vi "test bench_FXP_Linear_controller_observer.vi"() -> ()   [LabVIEW 2017]
uses:
  fixed-point/typeDefs/FXPControlParams_distEst.ctl
  fixed-point/typeDefs/x_vec_bram.ctl
  fixed-point/typeDefs/Kz_bram.ctl
  fixed-point/typeDefs/Nx_bram.ctl
  fixed-point/typeDefs/A_as_vec_bram.ctl
  fixed-point/typeDefs/Bz_bram.ctl
  fixed-point/typeDefs/Lz_bram.ctl
  <vilib>/rvi/DataTransferAndStorage/Container/Common/niFpgaContainerExecOnDevCompGetState.vi
  <vilib>/rvi/Emulation/niFpgaEmulationIsFPGAContextNoSignature.vi
  <vilib>/rvi/DataTransferAndStorage/Container/Common/niFpgaContainerGetUniqueNameForEmu.vi
  <vilib>/rvi/Emulation/niFpgaProcessEmulError.vi
  <vilib>/rvi/Emulation/niFpgaSctlEmulationGetInTimedLoop.vi
  <vilib>/rvi/errors/nirviReportUnexpectedCaseInternalError (U32).vi
  <vilib>/rvi/Memory/Memory_Emulation/niFpgaMemoryEmulationCacheClearOnFirstRun.vi
  <vilib>/rvi/Memory/Memory_Emulation/nirvimemoryEmulationManagerCache_MakeExclusive.vi
  <vilib>/rvi/Memory/Memory_Emulation/niFpgaMemoryEmulationValidateCache.vi
  <vilib>/rvi/Memory/Memory_Emulation/nirvimemoryEmulationManagerCache_InsertValue.vi
  <vilib>/Utility/error.llb/Clear Errors.vi
  <vilib>/rvi/Memory/Memory_Emulation/nirvimemoryEmulationManagerCache_ReleaseExclusive.vi
  <vilib>/rvi/Memory/Memory_Emulation/nirvimemoryEmulationManagerCache_GetValue.vi
  <vilib>/rvi/Memory/Memory_Emulation/nirvimemoryEmulationManagerCache_SetValue.vi
  <vilib>/rvi/Emulation/niFpgaSctlEmulationResourceMgr.vi
  <vilib>/rvi/DataTransferAndStorage/Container/XNode/niFpgaContainer.xnode
  <vilib>/rvi/Memory/Memory_Emulation/niFpgaMemoryEmulationRefIn.vi
panel:
  out "A*x":fxp<+/-,32,7>[](array[numeric]) format="%_10g"
  in  "matrix data":T1={"Bz"=[0.0, 0.0, 0.0, 0.0, 0.0, 0.0, 0.0, 0.0, 0.0, 0.0, 0.0, 0.0, 0.0, 0.0, 0.0, 0.0, 0.0, 0.0, 0.0, 0.0, 0.0, 0.0, 0.0, 0.0, 0.0, 0.0, 0.0, 0.0, 0.0, 0.0, 0.0, 0.0, 0.0, 0.0, 0.0, 0.0, 0.0, 0.0, 0.0, 0.0, 0.0, 0.0, 0.0, 0.0, 0.0, 0.0, 0.0, 0.0, 0.0, 0.0], "Ldist"=[-0.0729738399386406, -0.004303865134716034, -0.057222433388233185, -0.10025020688772202, -0.047570884227752686, -0.09535523504018784, -0.04109501093626022, -0.10293065756559372, -0.08871345221996307, -0.10357048362493515, -0.03105459362268448, -0.09562776982784271, 0.0, 0.0, 0.0, 0.0, 0.0, 0.0, 0.0, 0.0, 0.0, 1.066809631884098, 0.0, 0.0, 0.0, 0.0, 0.0, 0.0, 0.0, 0.0, 0.0, 0.0, 0.0, 0.0, 0.0, 0.0, 0.0, 0.0, 0.0, 0.0, 0.0, 0.0, 0.0, 0.0, 0.0, 0.0, 0.0, 0.0, 0.0, 0.0], "Kz"=[0.0150146484375, -0.01029205322265625, -0.00801849365234375, 166.71977996826172, 0.9633712768554688, -533.0425186157227, 252.25917053222656, 8929.314598083496, -5151.056785583496, -4194.612159729004, 784.6275939941406, -267.9263153076172, -1.0179214477539062, -0.41944122314453125, 0.15653228759765625, 0.68121337890625, 1.1305160522460938, 1.485992431640625, 1.7357406616210938, 1.8747711181640625, -0.26526641845703125, 0.6280746459960938, 0.0, 0.0, 0.0, 0.0, 0.0, 0.0, 0.0, 0.0, 0.0, 0.0, 0.0, 0.0, 0.0, 0.0, 0.0, 0.0, 0.0, 0.0, 0.0, 0.0, 0.0, 0.0, 0.0, 0.0, 0.0, 0.0, 0.0, 0.0], "Nx"=[0.10000000149011612, 0.10000000149011612, 0.10000000149011612, 0.10000000149011612, 0.10000000149011612, 0.10000000149011612, 0.10000000149011612, 0.10000000149011612, 0.10000000149011612, 0.10000000149011612, 0.10000000149011612, 0.10000000149011612, 0.10000000149011612, 0.10000000149011612, 0.10000000149011612, 0.10000000149011612, 0.10000000149011612, 0.10000000149011612, 0.10000000149011612, 0.10000000149011612, 0.10000000149011612, 1.4164387583732605, 0.0, 0.0, 0.0, 0.0, 0.0, 0.0, 0.0, 0.0, 0.0, 0.0, 0.0, 0.0, 0.0, 0.0, 0.0, 0.0, 0.0, 0.0, 0.0, 0.0, 0.0, 0.0, 0.0, 0.0, 0.0, 0.0, 0.0, 0.0], "Ax_col"=[1.3538216352462769, 0.3759167492389679, 0.0, 0.0, 0.0, 0.0, 0.0, 0.0, 0.0, 0.0, 0.0, 0.0, 0.0, 0.0, 0.0, 0.0, 0.0, 0.0, 0.0, 0.0, 0.0, 0.0729738399386406, -0.2026936039328575, 0.8613702282309532, 0.20541855692863464, -0.3512432351708412, 0.5301867201924324, 0.0, 0.0, 0.0, 0.0, 0.0, 0.0, 0.0, 0.0, 0.0, 0.0, 0.0, 0.0, 0.0, 0.0, 0.0, 0.0, 0.004303865134716034, 0.3965185433626175, 0.17570575326681137, 0.9175389409065247, -0.16186054050922394, 0.24432159960269928, 0.0, 0.0, 0.0, 0.0, 0.0, 0.0, 0.0, 0.0, 0.0, 0.0, 0.0, 0.0, 0.0, 0.0, 0.0, 0.0, 0.0, 0.0, 0.0, 0.0, 0.0, 0.0, 0.0, 0.0, 0.0, 0.0, 0.0, 0.0, 0.0, 0.0, 0.0, 0.0, 0.0, 0.0, 0.0, 0.0, 0.0, 0.0, 0.0, 0.0, 0.0, 0.0, 0.0, 0.0, 0.0, 0.0, 0.0, 0.0, 0.0, 0.0, 0.0, 0.0, 0.0, 0.0, 0.0, 0.0, 0.0, 0.0, 0.0, 0.0, 0.0, 0.0, 0.0, 0.0, 0.0, 0.0, 0.0, 0.0, 0.0, 0.0, 0.0, 0.0, 0.0, 0.0, 0.0, 0.0, 0.0, 0.0, 0.0, 0.0, 0.0, 0.0, 0.0, 0.0, 0.0, 0.0, 0.0, 0.0, 0.0, 0.0, 0.0, 0.0, 0.0, 0.0, 0.0, 0.0, 0.0, 0.0, 0.0, 0.0, 0.0, 0.0, 0.0, 0.0, 0.0, 0.0, 0.0, 0.0, 0.0, 0.0, 0.0, 0.0, 0.0, 0.0, 0.0, 0.0, 0.0, 0.0, 0.0, 0.0, 0.0, 0.0, 0.0, 0.0, 0.0, 0.0, 0.0, 0.0, 0.0, 0.0, 0.0, 0.0, 0.0, 0.0, 0.0, 0.0, 0.0, 0.0, 0.0, 0.0, 0.0, 0.0, 0.0, 0.0, 0.0, 0.0, 0.0, 0.0, 0.0, 0.0, 0.0, 0.0, 0.0, 0.0, 0.0, 0.0, 0.0, 0.0, 0.0, 0.0, 0.0, 0.0, 0.0, 0.0, 0.0, 0.0, 0.0, 0.0, 0.0, 0.0, 0.0, 0.0, 0.0, 0.0, 0.0, 0.0, 0.0, 0.0, 0.0, 0.0, 0.0, 0.0, 0.0, 0.0, 0.0, 0.0, 0.0, 0.0, 0.0, 0.0, 0.0, 0.0, 0.0, 0.0, 0.0, 0.0, 0.0, 0.0, 0.0, 0.0, 0.0, 0.0, 0.0, 0.0, 0.0, 0.0, 0.0, 0.0, 0.0, 0.0, 0.0, 0.0, 0.0, 0.0, 0.0, 0.0, 0.0, 0.0, 0.0, 0.0, 0.0, 0.0, 0.0, 0.0, 0.0, 0.0, 0.0, 0.0, 0.0, 0.0, 0.0, 0.0, 0.0, 0.0, 0.0, 0.0, 0.0, 0.0, 0.0, 0.0, 0.0, 0.0, 0.0, 0.0, 0.0, 0.0, 0.0, 0.0, 0.0, 0.0, 0.0, 0.0, 0.0, 0.0, 0.0, 0.0, 0.0, 0.0, 0.0, 0.0, 0.0, 0.0, 0.0, 0.0, 0.0, 0.0, 0.0, 0.0, 0.0, 0.0, 0.0, 0.0, 0.0, 0.0, 0.0, 0.0, 0.0, 0.0, 0.0, 0.0, 0.0, 0.0, 0.0, 0.0, 0.0, 0.0, 0.0, 0.0, 0.0, 0.0, 0.0, 0.0, 0.0, 0.0, 0.0, 0.0, 0.0, 0.0, 0.0, 0.0, 0.0, 0.0, 0.0, 0.0, 0.0, 0.0, 0.0, 0.0, 0.0, 0.0, 0.0, 0.0, 0.0, 0.0, 0.0, 0.0, 0.0, 0.0, 0.0, 0.0, 0.0, 0.0, 0.0, 0.0, 0.0, 0.0, 0.0, 0.0, 0.0, 0.0, 0.0, 0.0, 0.0, 0.0, 0.0, 0.0, 0.0, 0.0, 0.0, 0.0, 0.0, 0.0, 0.0, 0.0, 0.0, 0.0, 0.0, 0.0, 0.0, 0.0, 0.0, 0.0, 0.0, 0.0, 0.0, 0.0, 0.0, 0.0, 0.0, 0.0, 0.0, 0.0, 0.0, 0.0, 0.0, 0.0, 0.0, 0.0, 0.0, 0.0, 0.0, 0.0, 0.0, 0.0, 0.0, 0.0, 0.0, 0.0, 0.0, 0.0, 0.0, 0.0, 0.0, 0.0, 0.0, 0.0, 0.0, 0.0, 0.0, 0.0, 0.0, 0.0, 0.0, 0.0, 0.0, 0.0, 0.0, 0.0, 0.0, 0.0, 0.0, 0.0, 0.0, 0.0, 0.0, 0.0, 0.0, 0.0, 0.0, 0.0, 0.0, 0.0, 0.0, 0.0, 0.0, 0.0, 0.0, 0.0, 0.0, 0.0, 0.0, 0.0, 0.0, 0.0, 0.0, 0.0, 0.0, 0.0, 0.0, 0.0, 0.0, 0.0, 0.0, 0.0, 0.0, 0.0, 0.0, 0.0, 0.0, 0.0, 0.0, 0.0, 0.0, 0.0, 0.0, 0.0, 0.0, 0.0, 0.0, 0.0, 0.0]}
  in  "xk_1_0":fxp<+/-,32,5>[](array[numeric])=[0.0, 0.0, 0.0, 0.0, 0.0, 0.0, 0.0, 0.0, 0.0, 0.0, 0.0, 0.0, 0.0, 0.0, 0.0, 0.0, 0.0, 0.0, 0.0, 0.0, 0.0, 0.0, 0.0, 0.0, 0.0, 0.0, 0.0, 0.0, 0.0, 0.0, 0.0, 0.0, 0.0, 0.0, 0.0, 0.0, 0.0, 0.0, 0.0, 0.0, 0.0, 0.0, 0.0, 0.0, 0.0, 0.0, 0.0, 0.0, 0.0, 0.0]
  out "xk_1_0 (out)":fxp<+/-,32,5>[](array[numeric])
  out "xk_1_1":fxp<+/-,32,5>[](array[numeric])
  out "xk_1_2":fxp<+/-,32,5>[](array[numeric])
  out "yd_est":fxp<+/-,32,5>
  in  "y(k-1)":fxp<+/-,18,5>
  in  "u(k-1)":fxp<+/-,18,5>
  in  "x_u(k)":fxp<+/-,32,8>
  out "xerr":fxp<+/-,32,5>[](array[numeric])
  out "del u(k)":fxp<+/-,64,15>
  out "u_k (saturated)":fxp<+/-,32,5>
  out "saturated?":bool
  in  "ControlParams_distEst":T2={"umax"=3.0, "NS"=0, "ref_f_VEC"=[0.0, 0.0], "Nu11_22"=[0.0, 0.0], "u0"=[0.0, 0.0]} {"ref_f_VEC" format="%#_9g"}
  in  "du_umax":fxp<+/-,18,5>
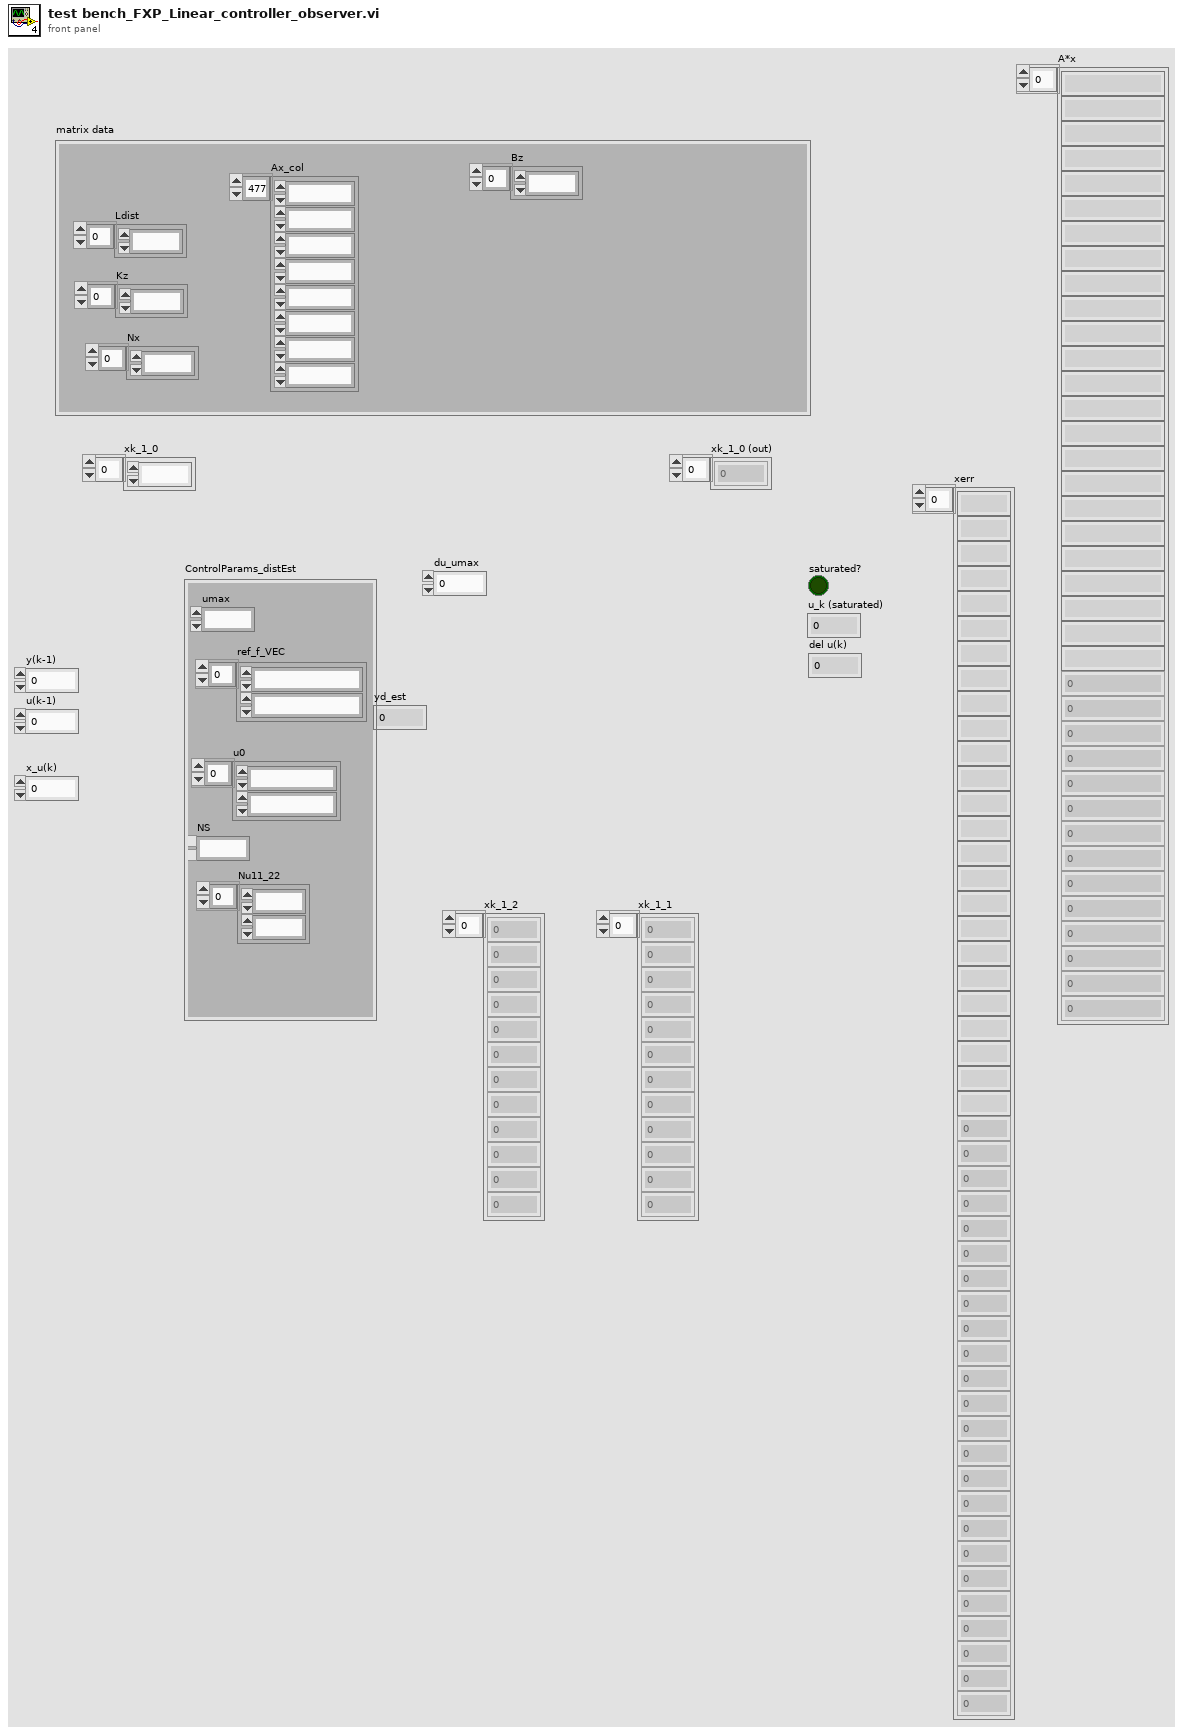
[diagram p1: front panel]
types:
  T1 = cluster{"Bz":fxp<+/-,32,5>[], "Ldist":fxp<+/-,32,5>[], "Kz":fxp<+/-,32,15>[], "Nx":fxp<+/-,32,5>[], "Ax_col":fxp<+/-,32,5>[]}
  T2 = typedef "FXPControlParams_distEst.ctl" = cluster{"umax":fxp<+/-,18,5>, "NS":u8, "ref_f_VEC":fxp<+/-,32,5>[], "Nu11_22":fxp<+/-,32,5>[], "u0":fxp<+/-,32,5>[]}
  T3 = typedef "x_vec_bram.ctl" = refnum<k21>
  T4 = typedef "Kz_bram.ctl" = refnum<k21>
  T5 = typedef "Nx_bram.ctl" = refnum<k21>
  T6 = typedef "A_as_vec_bram.ctl" = refnum<k21>
  T7 = typedef "Bz_bram.ctl" = refnum<k21>
  T8 = typedef "Lz_bram.ctl" = refnum<k21>
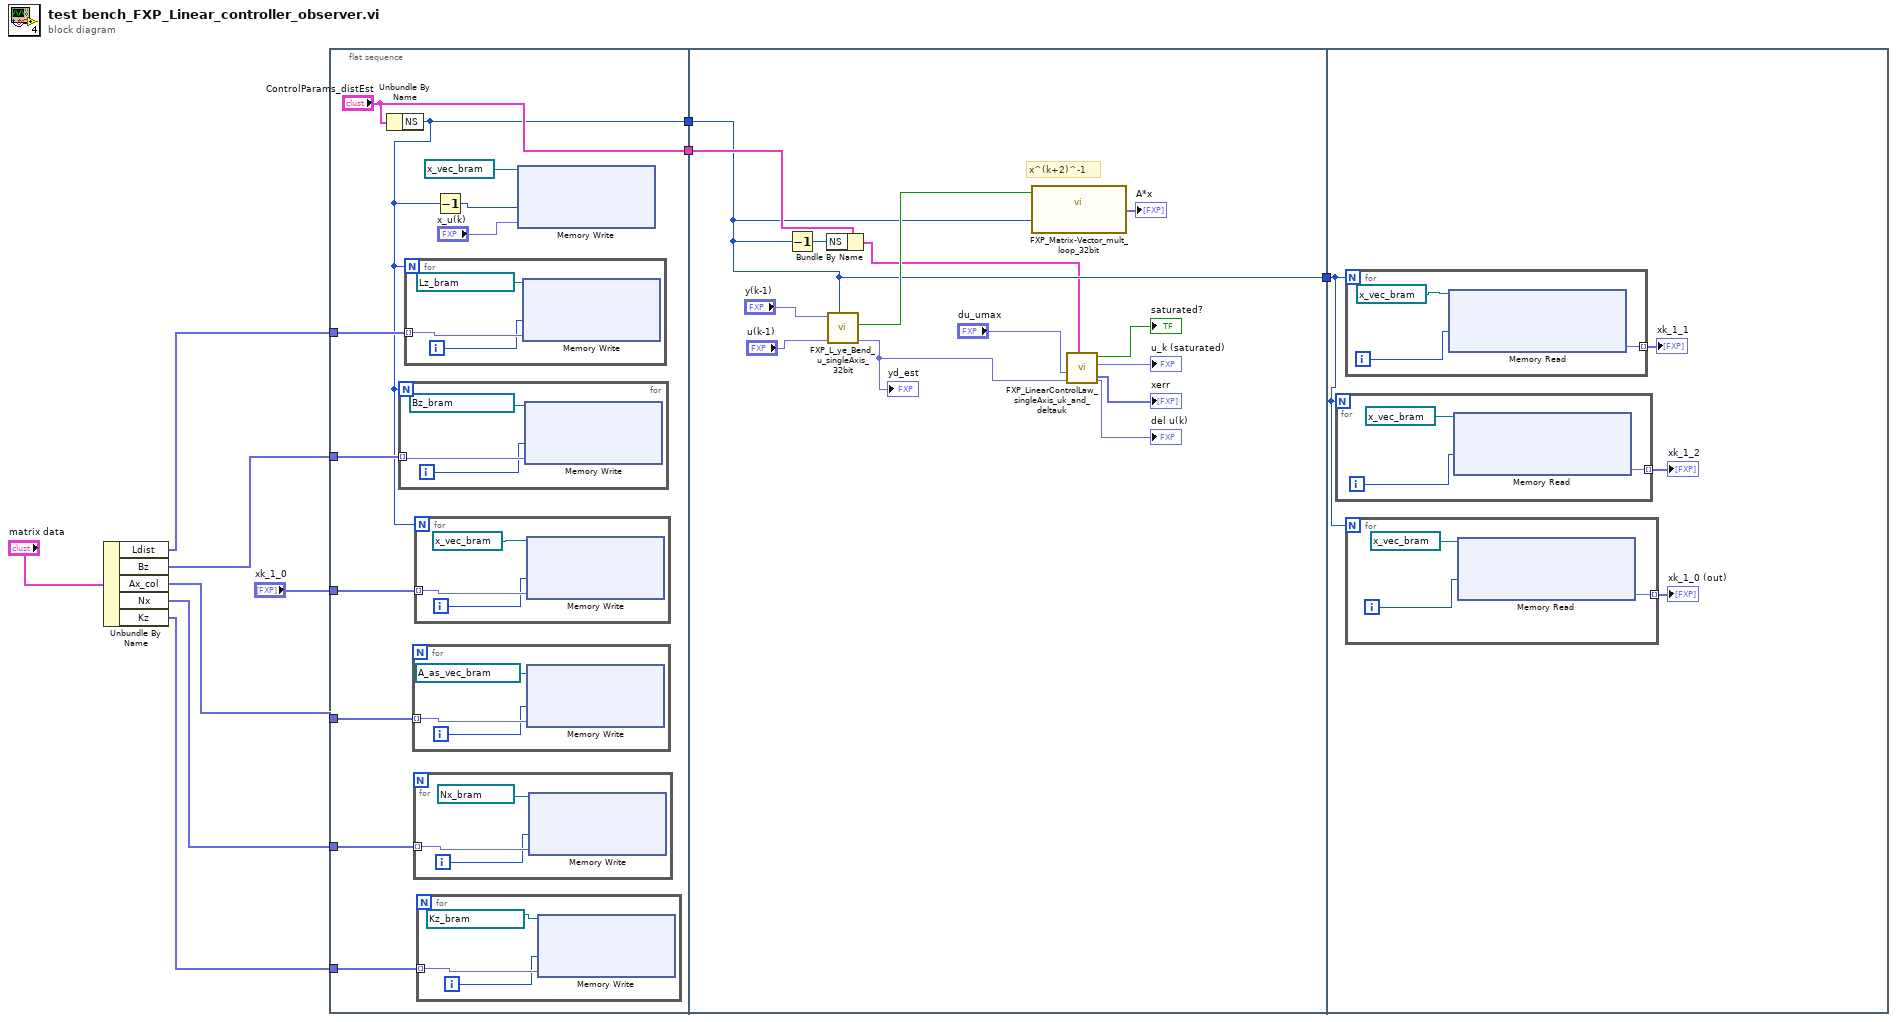
[diagram p0: block diagram]
diagram:
  n1 = Unbundle By Name("matrix data") -> ("Ldist"=w3:fxp<+/-,32,5>[], "Bz"=w2:fxp<+/-,32,5>[], "Ax_col"=w5:fxp<+/-,32,5>[], "Nx"=w4:fxp<+/-,32,5>[], "Kz"=w1:fxp<+/-,32,15>[])
  n2 = flat-sequence {
    tunnel: w3 -> [w21]
    tunnel: "xk_1_0" -> [w20]
    tunnel: w2 -> [w19]
    tunnel: ["ControlParams_distEst"] -> w9
    tunnel: [w15] -> w8
    tunnel: w5 -> [w14]
    tunnel: w4 -> [w13]
    tunnel: w1 -> [w12]
    tunnel: [w42] -> w10
    tunnel: w9 -> [w44]
    tunnel: w8 -> [w42]
    tunnel: w10 -> [w54]
    frame #0 {
      n3 = Unbundle By Name("ControlParams_distEst") -> ("NS"=w15:u8)
      n4 = for {
        N: w15 -> [_]
        tunnel: w19 -> [w36] mode=indexing
        i -> [w35]
        n5 = xnode "Memory Write"("Address"=w35, "Data"=w36, "Memory In"=T7 "Bz_FXP_col1" ("Memory")) -> ()  [unwired: 1 out]
      }
      n6 = for {
        N: w15 -> [_]
        tunnel: w21 -> [w39] mode=indexing
        i -> [w38]
        n7 = xnode "Memory Write"("Address"=w38, "Data"=w39, "Memory In"=T8 "L_FXP_col1" ("Memory")) -> ()  [unwired: 1 out]
      }
      n8 = for {
        tunnel: w14 -> [w30] mode=indexing
        i -> [w29]
        n9 = xnode "Memory Write"("Address"=w29, "Data"=w30, "Memory In"=T6 "AasCol _FXP") -> ()  [unwired: 1 out]
      }
      n10 = for {
        tunnel: w13 -> [w27] mode=indexing
        i -> [w26]
        n11 = xnode "Memory Write"("Address"=w26, "Data"=w27, "Memory In"=T5 "Nx_col1" ("Nx")) -> ()  [unwired: 1 out]
      }
      n12 = for {
        N: w15 -> [_]
        tunnel: w20 -> [w33] mode=indexing
        i -> [w32]
        n13 = xnode "Memory Write"("Address"=w32, "Data"=w33, "Memory In"=T3 "xk_1_0" ("Memory")) -> ()  [unwired: 1 out]
      }
      n14 = for {
        tunnel: w12 -> [w24] mode=indexing
        i -> [w23]
        n15 = xnode "Memory Write"("Address"=w23, "Data"=w24, "Memory In"=T4 "K_FXP_row1" ("Memory")) -> ()  [unwired: 1 out]
      }
      n16 = Decrement(x=w15) -> (x-1=w17:u8)
      n17 = xnode "Memory Write"("Address"=w17, "Data"="x_u(k)", "Memory In"=T3 "xk_1_2" ("Memory")) -> ()  [unwired: 1 out]
    }
    frame #1 {
      # "x^(k+2)^-1"
      n18 = Decrement(x=w42) -> (x-1=w43:u8)
      n19 = Bundle By Name(cluster=w44, "NS"=w43) -> (w41:T2)
      n20 = call "FXP_L_ye_Bend_u_singleAxis_32bit.vi"("NS"=w42, "U(k): ux"="u(k-1)", "Y(k): x"="y(k-1)") -> ("yd_est"=w45:fxp<+/-,32,5>, "outputValid"=w51:bool)  [unwired: 6 in, 1 out]
      "yd_est" <- w45
      n21 = call "FXP_Matrix-Vector_mult_loop_32bit.vi"("Ns_2"=w42, "inputValid"=w51) -> ("Array"=→"A*x":fxp<+/-,32,13>[])  [unwired: 9 in]
      n22 = call "FXP_LinearControlLaw_singleAxis_uk_and_deltauk.vi"("ControlParams_distEst"=w41, "yd_est_x"=w45, "du_max"="du_umax") -> ("del u_x"=→"del u(k)":fxp<+/-,64,15>, "u_k (saturated)"=→"u_k (saturated)":fxp<+/-,32,5>, "saturated?"=→"saturated?":bool, "xerr"=→"xerr":fxp<+/-,32,5>[])  [unwired: 5 in]
    }
    frame #2 {
      n23 = for {
        N: w54 -> [_]
        tunnel: [w62] -> w56 mode=indexing
        i -> [w63]
        n24 = xnode "Memory Read"("Address"=w63, "Memory In"=T3 "xk_1_2" ("Memory")) -> ("Data"=w62:fxp<+/-,32,6>)  [unwired: 1 out]
      }
      "xk_1_2" <- w56
      n25 = for {
        N: w54 -> [_]
        tunnel: [w65] -> w57 mode=indexing
        i -> [w66]
        n26 = xnode "Memory Read"("Address"=w66, "Memory In"=T3 "xk_1_1" ("Memory")) -> ("Data"=w65:fxp<+/-,32,6>)  [unwired: 1 out]
      }
      "xk_1_1" <- w57
      n27 = for {
        N: w54 -> [_]
        tunnel: [w59] -> w55 mode=indexing
        i -> [w60]
        n28 = xnode "Memory Read"("Address"=w60, "Memory In"=T3 "xk_1_0" ("Memory")) -> ("Data"=w59:fxp<+/-,32,6>)  [unwired: 1 out]
      }
      "xk_1_0 (out)" <- w55
    }
  }
